vi "Results search.vi"(11 "Path":path) -> (1 "Fail Item":string, 2 "Index of fail item":i32, 3 "p/f":bool)   [LabVIEW 2012]
uses:
  <vilib>/Utility/file.llb/Read From Spreadsheet File (string).vi
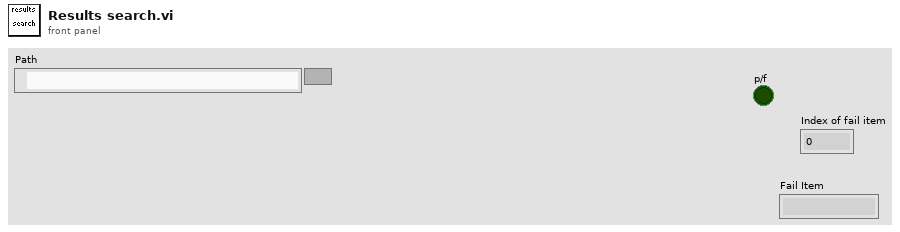
[diagram p1: front panel]
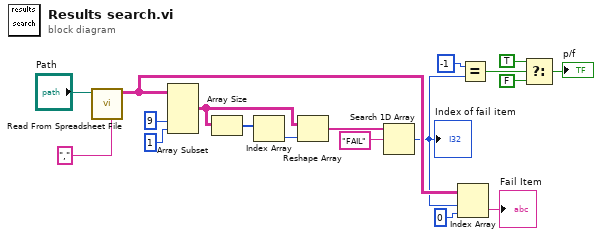
[diagram p0: block diagram]
diagram:
  n1 = call-poly <vilib>:"Read From Spreadsheet File.vi"("delimiter (\\t)"="," ("delimiter (\\t)"), "file path (dialog if empty)"="Path") -> ("all rows"=w4:string[][])  [unwired: 5 in, 4 out]
  n2 = Array Subset(array=w4, index (col)=9 ("index"), length (col)=1 ("length")) -> (w11:string[][])  [unwired: 2 in]
  n3 = Array Size(array=w11) -> (size(s)=w12:i32[])
  n4 = Index Array(array=w12) -> (element=w13:i32)  [unwired: 1 in]
  n5 = Reshape Array(w11, w13) -> (w14:string[])
  n6 = Search 1D Array(1D array=w14, element="FAIL") -> (index of element=w3:i32)  [unwired: 1 in]
  "Index of fail item" <- w3
  n7 = Index Array(array=w4, index (row)=w3, index (col)=0 ("disabled index (col)")) -> (element=→"Fail Item":string)
  n8 = Equal?(x=-1, y=w3) -> (x = y?=w17:bool)
  n9 = Select(t=TRUE, s=w17, f=FALSE) -> (s? t:f=→"p/f":bool)
